vi "command engine update FIFOs after responses.vi"(8 "error out":errorcluster, 9 "State Variables in":T18, 10 "Settings in":T1 {"Compiled"."External Channels"."Channels" format="%.0x"; "Compiled"."External Channels"."Triggers" format="%.0x"}, 11 "Global Variables in":T14) -> (0 "error out":errorcluster, 1 "State Variables out":T18, 2 "Settings out":T1 {"Compiled"."External Channels"."Channels" format="%.0x"; "Compiled"."External Channels"."Triggers" format="%.0x"}, 3 "Global Variables out":T14)   [LabVIEW 2018, in "Instrument Addon Engine.lvlib"]
uses:
  Instrument Addon Engine.lvlib
  <vilib>/NI/NIVS Inline Async API/_Data Access Engine/Data Access Engine/Data Access Engine.lvclass
  <vilib>/NI/NIVS Inline Async API/_Data Access Engine/Data Access Engine/Methods/Write.Data.vi
  <vilib>/NI/Tools/Keyed Array/KeyedArray.ctl
  <vilib>/NI/Tools/Keyed Array/Tools_KeyedArray.lvlib
  <vilib>/NI/AMC/Message.ctl
  <vilib>/NI/AMC/AMC.lvlib
  <vilib>/NI/AMC/Message Queue.ctl
  Types/Engine State Variables.ctl
  Addon Shared/Types/Linked Channel Cluster.ctl
  Addon Shared/Instrument Addon Shared.lvlib
  Addon Shared/Types/Command Parameters.ctl
  <vilib>/NI VeriStand/Custom Device API/Data Reference.ctl
  <vilib>/NI VeriStand/Custom Device API/Custom Device API.lvlib
  Addon Shared/Types/Response Wait Type.ctl
  Addon Shared/Types/Response Parameters.ctl
  Addon Shared/Types/Response RT Configuration Cluster.ctl
  Addon Shared/Types/Message Generation Type.ctl
  Addon Shared/Types/Message Parameters.ctl
  Types/Commands RT Configuration Cluster.ctl
  Types/command engine global variables.ctl
  Addon Shared/Types/External Trigger Refs.ctl
  Addon Shared/Types/Compiled Settings.ctl
  Source/Addon/Support Libraries/Protections.lvlibp/Parent Protection/Protection.lvclass
  Source/Addon/Support Libraries/Protocols.lvlibp/Protocol Parent/Protocol Parent.lvclass
  <vilib>/NI/NIVS Inline Async API/_VS Inline Async API/Process/Process.lvclass
  <vilib>/NI/NIVS Inline Async API/_Data Access Engine/Access Type Classes/ReadWrite/ReadWrite.lvclass
  <vilib>/NI/NI VeriStand Addon Network Comm/Engine/VeriStand Comm.lvclass
  <vilib>/NI/NIVS Inline Async API/_Data Access Engine/Access Type Classes/Write/Write.lvclass
  <vilib>/NI/NIVS Inline Async API/_Data Access Engine/Data Access Engine/Types/Write.DVR.ctl
  <vilib>/NI/NIVS Inline Async API/_Data Access Engine/Access Type Classes/Read/Read.lvclass
  <vilib>/NI/NIVS Inline Async API/_Data Access Engine/Data Access Engine/Types/Read.DVR.ctl
  <vilib>/NI/NIVS Inline Async API/_Data Access Engine/Data Access Engine/Types/ReadWrite.DVR.ctl
  Addon Shared/Types/Command Channel Index.ctl
  Addon Shared/Types/Command Channel Indeces.ctl
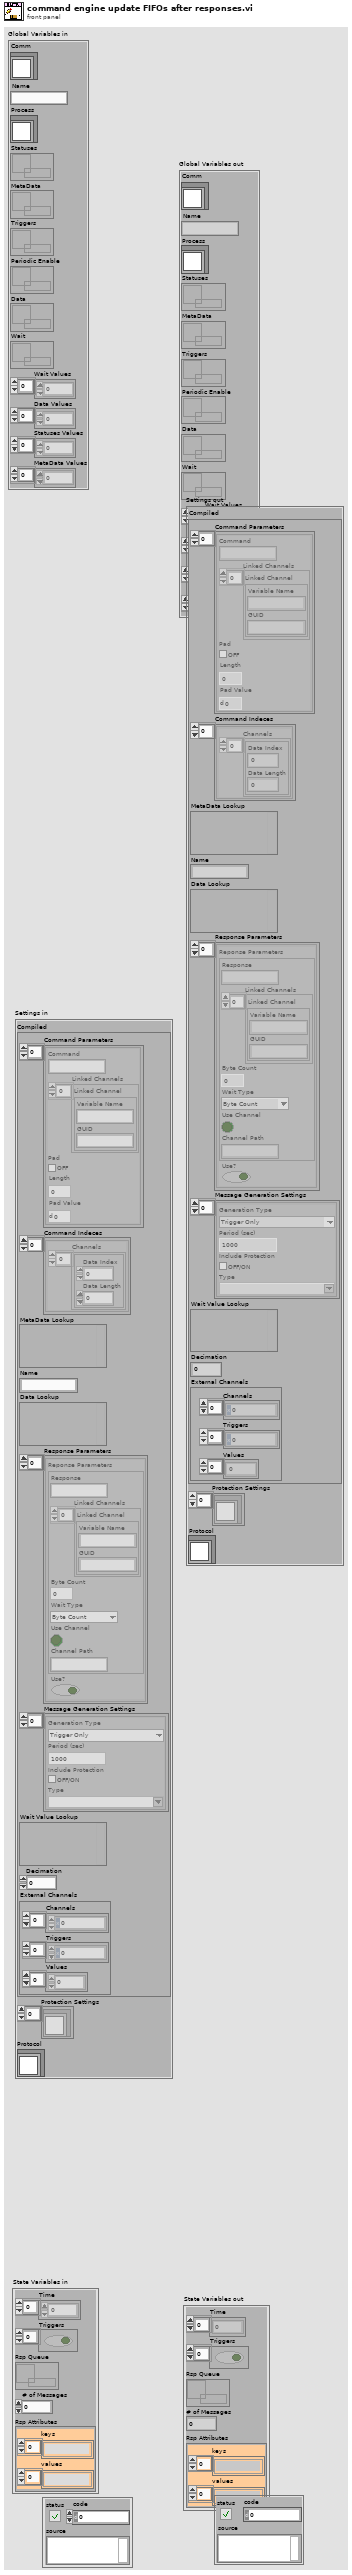
[diagram p1: front panel]
types:
  T1 = typedef "Instrument Addon Engine.lvlib/Commands RT Configuration Cluster.ctl" = cluster{"Compiled":T2, "Protection Settings":refnum<class "Protection.lvclass">[], "Protocol":refnum<class "Protocol Parent.lvclass">}
  T2 = typedef "Instrument Addon Shared.lvlib/Compiled Settings.ctl" = cluster{"Command Parameters":T3[], "Command Indeces":T5[], "MetaData Lookup":variant, "Name":string, "Data Lookup":variant, "Response Parameters":T7[], "Message Generation Settings":T10[], "Wait Value Lookup":variant, "Decimation":u32, "External Channels":T12}
  T3 = typedef "Instrument Addon Shared.lvlib/Command Parameters.ctl" = cluster{"Command":string, "Linked Channels":T4[], "Pad":bool, "Length":u32, "Pad Value":u8}
  T4 = typedef "Instrument Addon Shared.lvlib/Linked Channel Cluster.ctl" = cluster{"Variable Name":string, "GUID":string}
  T5 = typedef "Instrument Addon Shared.lvlib/Command Channel Indeces.ctl" = cluster{"Channels":T6[]}
  T6 = typedef "Instrument Addon Shared.lvlib/Command Channel Index.ctl" = cluster{"Data Index":i32, "Data Length":i32}
  T7 = typedef "Instrument Addon Shared.lvlib/Response RT Configuration Cluster.ctl" = cluster{"Reponse Parameters":T8, "Use?":bool}
  T8 = typedef "Instrument Addon Shared.lvlib/Response Parameters.ctl" = cluster{"Response":string, "Linked Channels":T4[], "Type Value":dbl, "Wait Type":T9, "Use Channel":bool, "Channel Path":string}
  T9 = typedef "Instrument Addon Shared.lvlib/Response Wait Type.ctl" = enum16{"Byte Count", "Wait sec"}
  T10 = typedef "Instrument Addon Shared.lvlib/Message Parameters.ctl" = cluster{"Generation Type":T11, "Period":dbl, "Include Protection":bool, "Type":string}
  T11 = typedef "Instrument Addon Shared.lvlib/Message Generation Type.ctl" = enum16{"Trigger Only", "Periodic & Trigger", "Value Change & Trigger"}
  T12 = typedef "Instrument Addon Shared.lvlib/External Trigger Refs.ctl" = cluster{"Channels":T13[], "Triggers":T13[], "Values":dbl[]}
  T13 = typedef "Custom Device API.lvlib/Data Reference.ctl" = i32
  T14 = typedef "Instrument Addon Engine.lvlib/Engine State Variables.ctl" = cluster{"Comm":refnum<class "VeriStand Comm.lvclass">, "Name":string, "Process":refnum<class "Process.lvclass">, "Statuses":T15, "MetaData":T16, "Triggers":T17, "Periodic Enable":T16, "Data":T15, "Wait":T16, "Wait Values":dbl[], "Data Values":dbl[], "Statuses Values":dbl[], "MetaData Values":dbl[]}
  T15 = typedef "Data Access Engine.lvlib/Data Access Engine.lvclass/Write.DVR.ctl" = refnum<data-value>
  T16 = typedef "Data Access Engine.lvlib/Data Access Engine.lvclass/Read.DVR.ctl" = refnum<data-value>
  T17 = typedef "Data Access Engine.lvlib/Data Access Engine.lvclass/ReadWrite.DVR.ctl" = refnum<data-value>
  T18 = typedef "Instrument Addon Engine.lvlib/command engine global variables.ctl" = cluster{"Time":u32[], "Triggers":bool[], "Rsp Queue":T19, "# of Messages":i32, "Rsp Attributes":T20}
  T19 = typedef "AMC.lvlib/Message Queue.ctl" = refnum<queue>
  T20 = typedef "Tools_KeyedArray.lvlib/KeyedArray.ctl" = cluster{"keys":string[], "values":string[]}
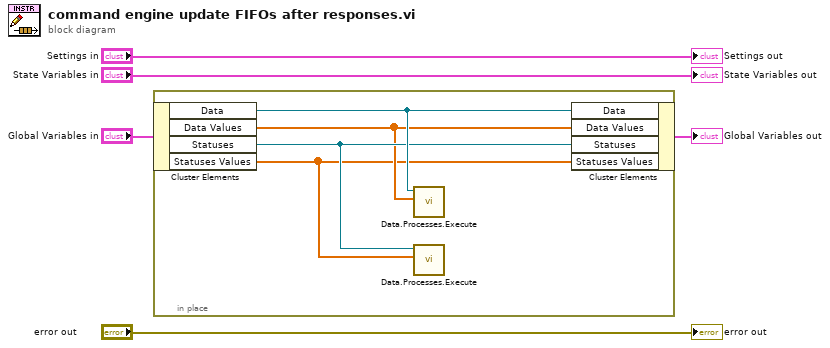
[diagram p0: block diagram]
diagram:
  n1 = in-place {
    n2 = in-place-cluster #1("Global Variables in") -> ("Data"=w9:T15, "Data Values"=w7:dbl[], "Statuses"=w8:T15, "Statuses Values"=w6:dbl[])
    n3 = call-poly <vilib>:"Data.Processes.Execute.vi"("Values"=w7, "Ref"=w9) -> ()  [unwired: 9 in, 1 out]
    n4 = call-poly <vilib>:"Data.Processes.Execute.vi"("Values"=w6, "Ref"=w8) -> ()  [unwired: 9 in, 1 out]
    n5 = in-place-cluster #1("Data"=w9, "Data Values"=w7, "Statuses"=w8, "Statuses Values"=w6) -> (→"Global Variables out":T14)
  }
  "Settings out" <- "Settings in"
  "State Variables out" <- "State Variables in"
  "error out" <- "error out"
